vi "TEST_bench_hysteresis_fxp_16_5.vi"(7 "N_hyst":i32, 11 "uk":sgl format="%#_13g") -> (3 "H_of_ik (expected)":sgl)   [LabVIEW 2017]
uses:
  <vilib>/Platform/TimedLoop/XDataNode/timing_clust.ctl
  <vilib>/Platform/TimedLoop/XDataNode/nitl_modes.ctl
  <vilib>/Platform/TimedLoop/XDataNode/wakeup.ctl
  <vilib>/rvi/Emulation/niFpgaSctlEmulationGetInTimedLoop.vi
  <vilib>/rvi/Emulation/niFpgaEmulationReportErrorSimple.vi
  <vilib>/rvi/Emulation/niFpgaGetClockAttributes.vi
  <vilib>/rvi/Emulation/niFpgaCriticalErrorInLSC.vi
  <vilib>/rvi/Memory/Memory_Emulation/nirvimemoryFastEmulation.vi
  <vilib>/rvi/Memory/Memory_Emulation/nirvimemoryEmulation.vi
  <vilib>/rvi/Emulation/niFpgaEmulationIsFPGAContextNoSignature.vi
  <vilib>/rvi/DataTransferAndStorage/Container/Common/niFpgaContainerGetUniqueNameForEmu.vi
  <vilib>/rvi/Emulation/niFpgaProcessEmulError.vi
  <vilib>/rvi/errors/nirviReportUnexpectedCaseInternalError (U32).vi
  <vilib>/Platform/TimedLoop/XDataNode/XDataNode.xnode
  <vilib>/rvi/DataTransferAndStorage/Container/XNode/niFpgaContainer.xnode
  <vilib>/Platform/TimedLoop/XDataNode/XDNodeRunTimeDep.lvlib
panel:
  out "y_vec_out (expected)":sgl[](array[numeric])
  out "y_out_mem":fxp<+/-,16,5>[](array[numeric])
  out "s 2":sgl
  in  "y_vec_in":fxp<+/-,16,5>[](array[numeric])=[0.0, 0.0, 0.0, 0.0, 0.0, 0.0, 0.0]
  in  "r_s":fxp<+/-,16,5>[](array[numeric])=[0.0, 0.0, 0.0, 0.0, 0.0, 0.0, 0.0]
  in  "w_s":fxp<+/-,16,5>[](array[numeric])=[0.0, 0.0, 0.0, 0.0, 0.0, 0.0, 0.0]
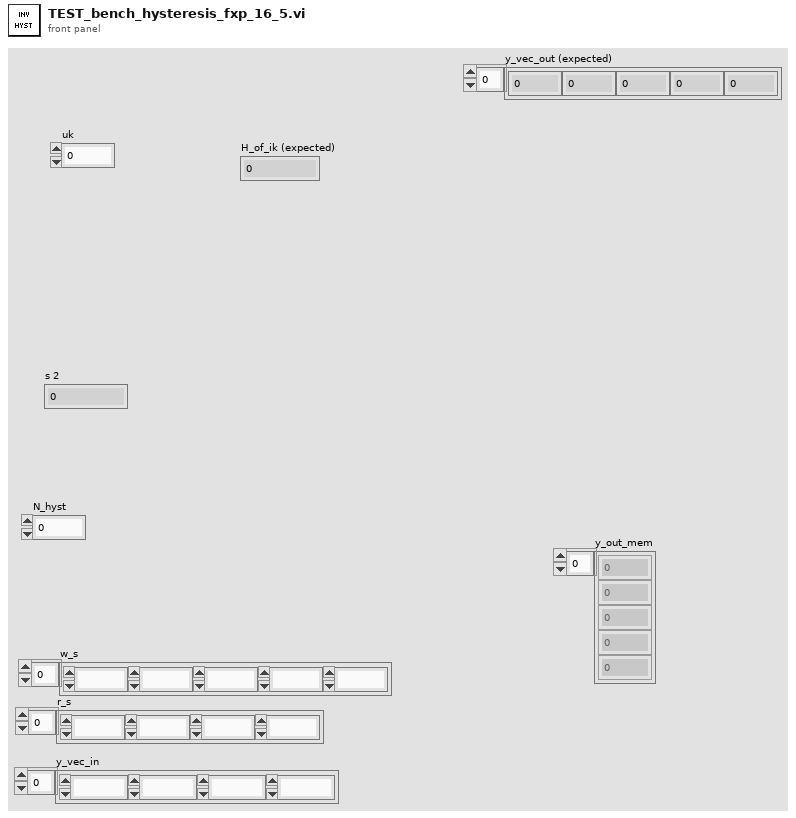
[diagram p1: front panel]
types:
  T1 = typedef "XDNodeRunTimeDep.lvlib/timing_clust.ctl" = cluster{"Expected End [f-1]":u64, "Actual End [f-1]":u64, "Finished Late? [f-1]":bool, "Expected End [i-1]":u64, "Actual End [i-1]":u64, "Finished Late? [i-1]":bool, "Expected Start [i]":u64, "Actual Start [i]":u64, "Expected Start [f]":u64, "Actual Start [f]":u64, "Source Name":string, "Structure Name":string, "Period":i64, "Deadline":i64, "Offset":i64, "Start":i64, "Priority":i32, "Timeout":i32, "Mode":T2, "Wakeup Reason":T3, "Error":errorcluster, "Source Type":string, "Secondary Source Type":string, "Global End Time":u64, "Global Start Time":u64, "Frame Duration":u64, "Iteration Duration":u64, "Assigned CPU":i32, "I/O Scan Engine Mode":u32}
  T2 = typedef "XDNodeRunTimeDep.lvlib/nitl_modes.ctl" = enum32{"No Change", "Process missed periods, maintain original phase", "Discard missed periods, maintain original phase", "Process missed periods, ignore original phase", "Discard missed periods, ignore original phase"}
  T3 = typedef "XDNodeRunTimeDep.lvlib/wakeup.ctl" = enum32{"Normal", "Aborted", "Asynchronous wakeup", "Timing source error", "Timed loop error", "Timeout"}
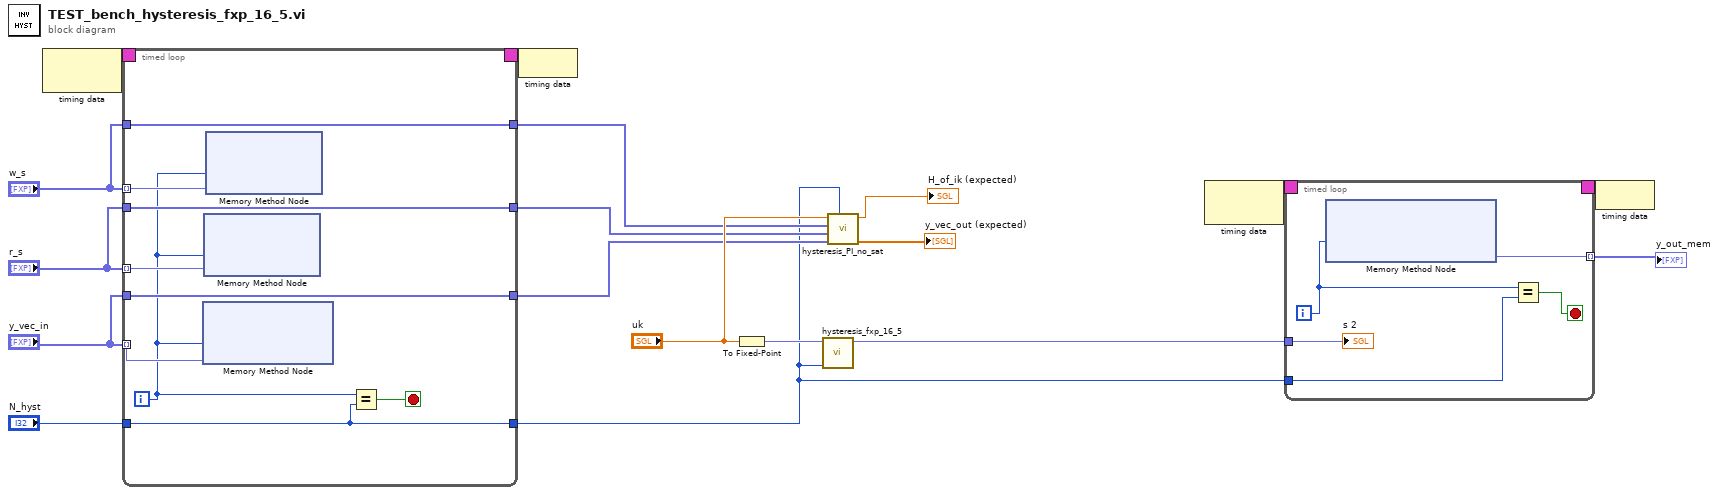
[diagram p0: block diagram]
diagram:
  n1 = node-c288() -> (w13:T1)  [unwired: 1 in]
  n2 = timed-loop {
    timing: w13 -> [_]
    timing-out: [_] -> w12
    tunnel: "w_s" -> [w26] mode=indexing
    tunnel: "r_s" -> [w24] mode=indexing
    tunnel: "y_vec_in" -> [w25] mode=indexing
    tunnel: [w23] -> w8
    tunnel: "w_s" -> [w23]
    tunnel: [w22] -> w7
    tunnel: "r_s" -> [w22]
    tunnel: [w21] -> w6
    tunnel: "y_vec_in" -> [w21]
    tunnel: "N_hyst" -> [w19]
    tunnel: [w19] -> w1
    i -> [w20]
    stop <- w27 stop-if-true
    n3 = xnode ("Memory Method Node")("Address"=w20, "Data"=w25) -> ()  [unwired: 1 in, 1 out]
    n4 = xnode ("Memory Method Node")("Address"=w20, "Data"=w24) -> ()  [unwired: 1 in, 1 out]
    n5 = xnode ("Memory Method Node")("Address"=w20, "Data"=w26) -> ()  [unwired: 1 in, 1 out]
    n6 = Equal?(x=w20, y=w19) -> (x = y?=w27:bool)
  }
  n7 = node-c288(w12) -> ()
  n8 = To Fixed-Point(number="uk") -> (fixed-point=w18:fxp<+/-,16,5>)  [unwired: 1 in]
  n9 = call "hysteresis_fxp_16_5.vi"("N_hyst"=w1, "uk_in"=w18) -> ("Hinv(uk)"=w14:fxp<+/-,32,10>)  [unwired: 9 in]
  n10 = call "hysteresis_PI_no_sat.vi"("N_hyst"=w1, "y_vec_in"=w6, "r_s"=w7, "w_s"=w8, "uk"="uk") -> ("y_vec_out"=→"y_vec_out (expected)":sgl[], "H_of_ik"=→"H_of_ik (expected)":sgl)  [unwired: 5 in]
  n11 = node-c288() -> (w17:T1)  [unwired: 1 in]
  n12 = timed-loop {
    timing: w17 -> [_]
    timing-out: [_] -> w16
    tunnel: [w34] -> w15 mode=indexing
    tunnel: w14 -> [w33]
    tunnel: w1 -> [w30]
    i -> [w31]
    stop <- w32 stop-if-true
    n13 = xnode ("Memory Method Node")("Address"=w31) -> ("Data"=w34:fxp<+/-,16,5>)  [unwired: 1 in, 1 out]
    n14 = Equal?(x=w31, y=w30) -> (x = y?=w32:bool)
    "s 2" <- w33
  }
  "y_out_mem" <- w15
  n15 = node-c288(w16) -> ()
